vi "ScanParameter.vi"(8 "error in (no error)":errorcluster, 11 "ScriptEditorV2 in":refnum<class "ScriptEditorV2.lvclass">) -> (0 "error out":errorcluster, 3 "ScriptEditorV2 out":refnum<class "ScriptEditorV2.lvclass">)   [LabVIEW 2009, in "Views.lvlib" / "ScriptEditor.lvlib" / "ScriptEditorV2.lvclass"]
uses:
  ScriptEditorV2.lvclass
  ScanCreator/ScanCreator.lvclass
  ScriptEditorV2.lvclass/ScriptEditorV2.ctl
  Tools/Scripting/ScriptingEvent/ScriptEventList/ScriptEventList.lvclass
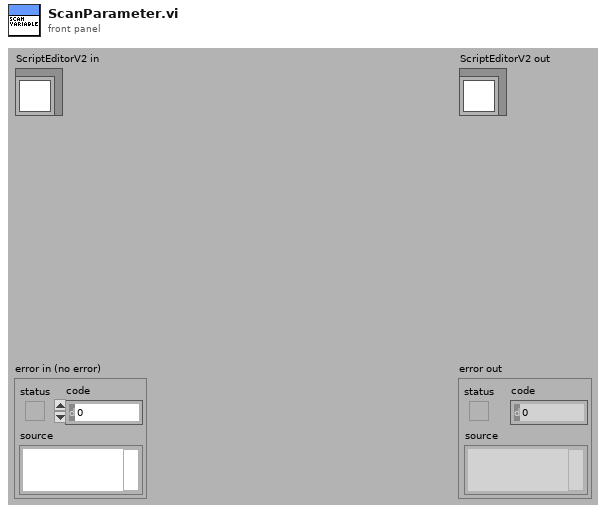
[diagram p1: front panel]
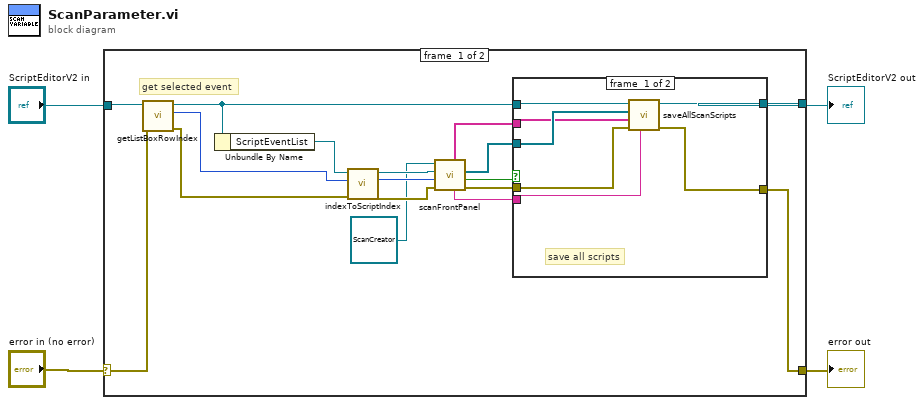
[diagram p0: block diagram]
diagram:
  n1 = case shown="No Error" "error in (no error)" {
    selector: "error in (no error)" -> [w18 w30]
    tunnel: [w9 w31] -> w3
    tunnel: "ScriptEditorV2 in" -> [w19 w31]
    tunnel: [w5 w30] -> w1
    frame #0 {
      # "get selected event"
      n2 = call "getListBoxRowIndex.vi"("error in (no error)"=w18, "ScriptEditorV2 in"=w19) -> ("error out"=w13:errorcluster, "rowIndex"=w21:i32, "ScriptEditorV2 out"=w10:refnum<class "ScriptEditorV2.lvclass">)  [unwired: 7 in]
      n3 = Unbundle By Name(w10) -> ("ScriptEventList"=w20:refnum<class "ScriptEventList.lvclass">)
      n4 = call "indexToScriptIndex.vi"("error in (no error)"=w13, "sequencedIndex"=w21, "ScriptEventList in"=w20) -> ("error out"=w15:errorcluster, "indexScriptEvent"=w16:i32, "ScriptEventList out"=w17:refnum<class "ScriptEventList.lvclass">)  [unwired: 6 in]
      n5 = call "scanFrontPanel.vi"("error in (no error)"=w15, "index"=w16, "ScriptEventList"=w17, "ScanCreator in"=refnum<class "ScanCreator.lvclass"> refnum) -> ("error out"=w6:errorcluster, "cancelled"=w12:bool, "scriptListArray"=w11:refnum<class "ScriptEventList.lvclass">[], "scanType"=w7:string, "Values"=w8:string[])  [unwired: 2 in, 1 out]
      n6 = case shown="False" w12 {
        tunnel: w11 -> [w24 _]
        tunnel: w10 -> [w28 w29]
        tunnel: [w26 w29] -> w9
        tunnel: w8 -> [w23 _]
        tunnel: w7 -> [w22 _]
        tunnel: w6 -> [w27 _]
        tunnel: [w25 _] -> w5
        frame #0 {
          # "save all scripts"
          n7 = call "saveAllScanScripts.vi"("scanType"=w22, "error in (no error)"=w27, "Values"=w23, "scriptListArray"=w24, "ScriptEditorV2 in"=w28) -> ("error out"=w25:errorcluster, "ScriptEditorV2 out"=w26:refnum<class "ScriptEditorV2.lvclass">)  [unwired: 5 in]
        }
        frame #1 {
          # "cancelled"
        }
      }
    }
    frame #1 {
    }
  }
  "error out" <- w1
  "ScriptEditorV2 out" <- w3
